vi "how_to_use.vi"() -> ()   [LabVIEW 2009]
panel:
  out "送信波形":cluster{dbl[], dbl[]}(graph)
  out "搬送波":cluster{dbl[], dbl[]}(graph)
  out "方形波":cluster{dbl[], dbl[]}(graph)
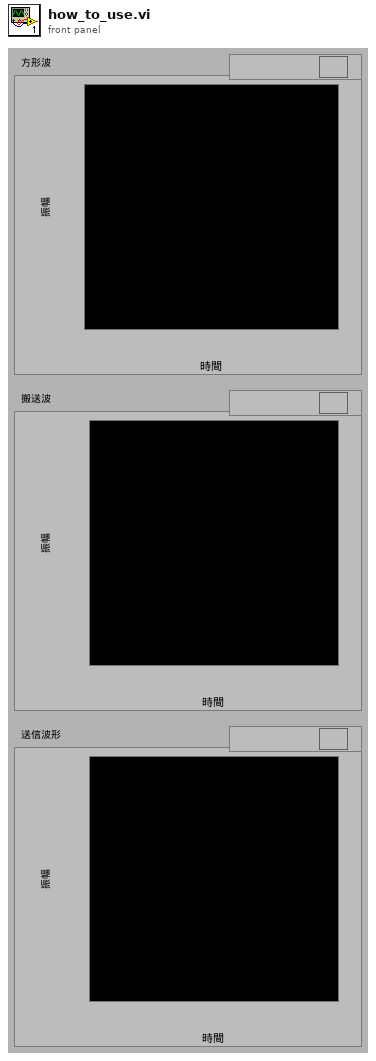
[diagram p1: front panel]
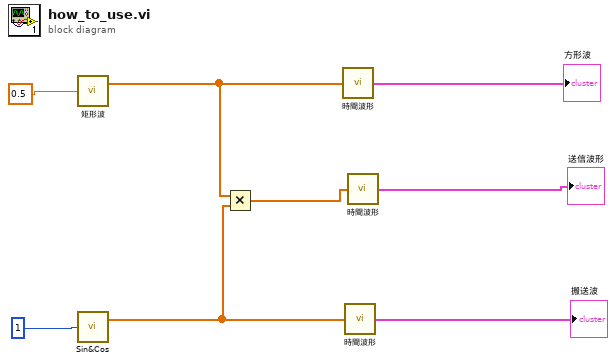
[diagram p0: block diagram]
diagram:
  n1 = call "矩形波.vi"("信号周波数 [kHz]"=0.5) -> ("矩形波"=w6:dbl[])  [unwired: 1 out]
  n2 = call "Sin&Cos.vi"("周波数[kHz]"=1) -> ("sin"=w7:dbl[])  [unwired: 1 out]
  n3 = Multiply(x=w6, y=w7) -> (x*y=w5:dbl[])
  n4 = call "時間波形.vi"("入力"=w6) -> ("時間波形"=→"方形波":cluster{dbl[], dbl[]})
  n5 = call "時間波形.vi"("入力"=w7) -> ("時間波形"=→"搬送波":cluster{dbl[], dbl[]})
  n6 = call "時間波形.vi"("入力"=w5) -> ("時間波形"=→"送信波形":cluster{dbl[], dbl[]})
